vi "True Pulse.vi"(11 "y":bool) -> (3 ".not. (x .or. y)?":bool)   [LabVIEW 2016]
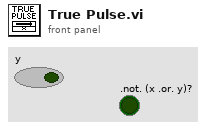
[diagram p1: front panel]
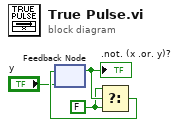
[diagram p0: block diagram]
diagram:
  w2 = FALSE ("y")
  n1 = feedback #1("y") -> (w4:bool)
  ".not. (x .or. y)?" <- w4
  n2 = Select(t=w2, s=w4, f=w2) -> (s? t:f=w3:bool)
  n3 = feedback-in #1(w3) -> ()
